vi "DIOs_ECD.vi"(0 "Mod6/DIOs":T1, 1 "Mod5/DIOs":T2) -> ()   [LabVIEW 2017]
uses:
  <vilib>/rvi/eio/common/nirviEmuTemplateMethod_errors.vi
  <vilib>/eio/EIONode/EIONode.xnode
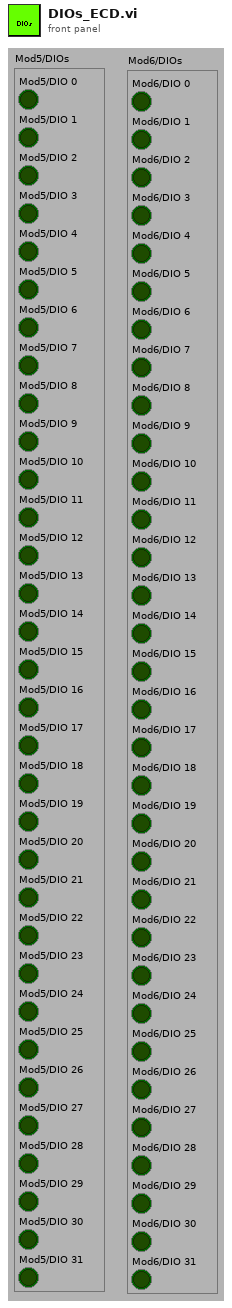
[diagram p1: front panel]
types:
  T1 = cluster{"Mod6/DIO 0":bool, "Mod6/DIO 1":bool, "Mod6/DIO 2":bool, "Mod6/DIO 3":bool, "Mod6/DIO 4":bool, "Mod6/DIO 5":bool, "Mod6/DIO 6":bool, "Mod6/DIO 7":bool, "Mod6/DIO 8":bool, "Mod6/DIO 9":bool, "Mod6/DIO 10":bool, "Mod6/DIO 11":bool, "Mod6/DIO 12":bool, "Mod6/DIO 13":bool, "Mod6/DIO 14":bool, "Mod6/DIO 15":bool, "Mod6/DIO 16":bool, "Mod6/DIO 17":bool, "Mod6/DIO 18":bool, "Mod6/DIO 19":bool, "Mod6/DIO 20":bool, "Mod6/DIO 21":bool, "Mod6/DIO 22":bool, "Mod6/DIO 23":bool, "Mod6/DIO 24":bool, "Mod6/DIO 25":bool, "Mod6/DIO 26":bool, "Mod6/DIO 27":bool, "Mod6/DIO 28":bool, "Mod6/DIO 29":bool, "Mod6/DIO 30":bool, "Mod6/DIO 31":bool}
  T2 = cluster{"Mod5/DIO 0":bool, "Mod5/DIO 1":bool, "Mod5/DIO 2":bool, "Mod5/DIO 3":bool, "Mod5/DIO 4":bool, "Mod5/DIO 5":bool, "Mod5/DIO 6":bool, "Mod5/DIO 7":bool, "Mod5/DIO 8":bool, "Mod5/DIO 9":bool, "Mod5/DIO 10":bool, "Mod5/DIO 11":bool, "Mod5/DIO 12":bool, "Mod5/DIO 13":bool, "Mod5/DIO 14":bool, "Mod5/DIO 15":bool, "Mod5/DIO 16":bool, "Mod5/DIO 17":bool, "Mod5/DIO 18":bool, "Mod5/DIO 19":bool, "Mod5/DIO 20":bool, "Mod5/DIO 21":bool, "Mod5/DIO 22":bool, "Mod5/DIO 23":bool, "Mod5/DIO 24":bool, "Mod5/DIO 25":bool, "Mod5/DIO 26":bool, "Mod5/DIO 27":bool, "Mod5/DIO 28":bool, "Mod5/DIO 29":bool, "Mod5/DIO 30":bool, "Mod5/DIO 31":bool}
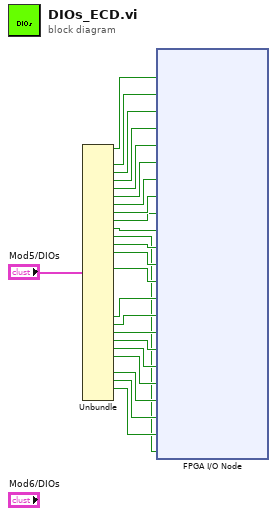
[diagram p0: block diagram]
diagram:
  n1 = Unbundle("Mod5/DIOs") -> ("Mod5/DIO 0"=w23:bool, "Mod5/DIO 2"=w22:bool, "Mod5/DIO 3"=w21:bool, "Mod5/DIO 4"=w20:bool, "Mod5/DIO 5"=w19:bool, "Mod5/DIO 6"=w18:bool, "Mod5/DIO 7"=w17:bool, "Mod5/DIO 8"=w16:bool, "Mod5/DIO 9"=w15:bool, "Mod5/DIO 10"=w14:bool, "Mod5/DIO 11"=w1:bool, "Mod5/DIO 12"=w13:bool, "Mod5/DIO 13"=w12:bool, "Mod5/DIO 15"=w11:bool, "Mod5/DIO 21"=w10:bool, "Mod5/DIO 22"=w9:bool, "Mod5/DIO 23"=w8:bool, "Mod5/DIO 24"=w7:bool, "Mod5/DIO 25"=w6:bool, "Mod5/DIO 26"=w5:bool, "Mod5/DIO 28"=w4:bool, "Mod5/DIO 29"=w3:bool, "Mod5/DIO 30"=w2:bool)  [unwired: 9 out]
  n2 = xnode "FPGA I/O Node"("Mod5/DIO0"=w23, "Mod5/DIO2"=w22, "Mod5/DIO3"=w21, "Mod5/DIO4"=w20, "Mod5/DIO5"=w19, "Mod5/DIO6"=w18, "Mod5/DIO7"=w17, "Mod5/DIO8"=w16, "Mod5/DIO9"=w15, "Mod5/DIO10"=w14, "Mod5/DIO12"=w13, "Mod5/DIO13"=w12, "Mod5/DIO15"=w11, "Mod5/DIO21"=w10, "Mod5/DIO22"=w9, "Mod5/DIO23"=w8, "Mod5/DIO24"=w7, "Mod5/DIO25"=w6, "Mod5/DIO26"=w5, "Mod5/DIO28"=w4, "Mod5/DIO29"=w3, "Mod5/DIO30"=w2, "Mod5/DIO11"=w1) -> ()  [unwired: 23 in, 23 out]
